vi "Read Buffer.vi"(8 "error in (no error)":errorcluster, 11 "Measure in":refnum<class "Measure.lvclass">) -> (0 "error out":errorcluster, 2 "Buffer":string, 3 "Measure out":refnum<class "Measure.lvclass">)   [LabVIEW 2023, in "HAF.lvlib" / "Measure.lvclass"]
uses:
  Measure.lvclass
  Measure.lvclass/Measure.ctl
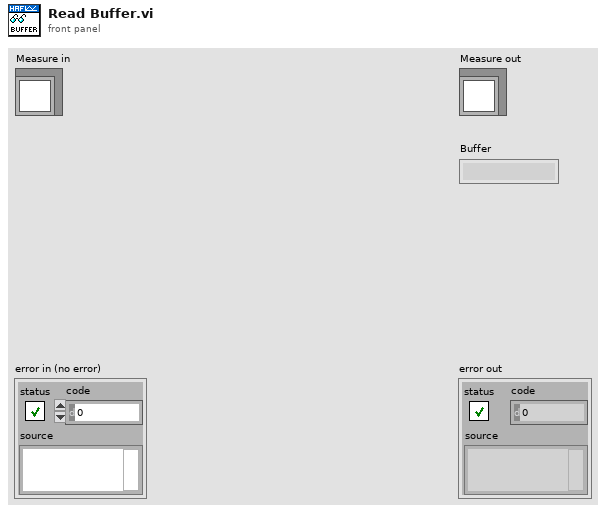
[diagram p1: front panel]
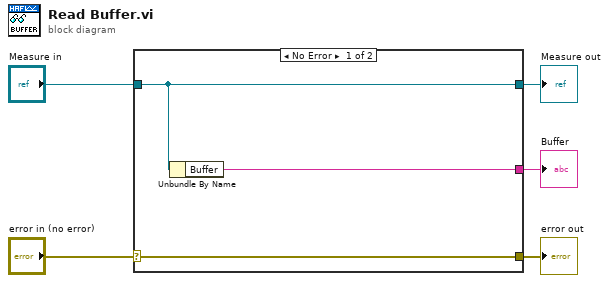
[diagram p0: block diagram]
diagram:
  n1 = case shown="No Error" "error in (no error)" {
    selector: "error in (no error)" -> [w8 w9]
    tunnel: [w8 w9] -> w4
    tunnel: [w7 w10] -> w2
    tunnel: "Measure in" -> [w7 w10]
    tunnel: [w6 _] -> w1
    frame No Error {
      n2 = Unbundle By Name(w7) -> ("Buffer"=w6:string)
    }
    frame Error {
    }
  }
  "error out" <- w4
  "Measure out" <- w2
  "Buffer" <- w1
